vi "putFPGAData.vi"(8 "error in (no error)":errorcluster, 10 "TelemetryFPGAData":T1, 11 "M1M3SAL in":refnum<class "M1M3SAL.lvclass">) -> (0 "error out":errorcluster, 3 "M1M3SAL out":refnum<class "M1M3SAL.lvclass">)   [LabVIEW 2016, in "M1M3SupportCommunicator.lvlib" / "M1M3SAL.lvclass"]
uses:
  M1M3SAL.lvclass
  DataTypes/Topics/TelemetryFPGAData.ctl
  DataTypes/Topics/Parts/Timestamp.ctl
  DataTypes/MessageHeader.ctl
  DataTypes/MessageTypes.ctl
  DataTypes/MessageTopics.ctl
  M1M3SAL.lvclass/M1M3SAL.ctl
  writeU8.vi
  writeI32.vi
  M1M3SupportCommunicator.lvlib
  DataTypes/Topics/M1M3SupportTopics.lvlib
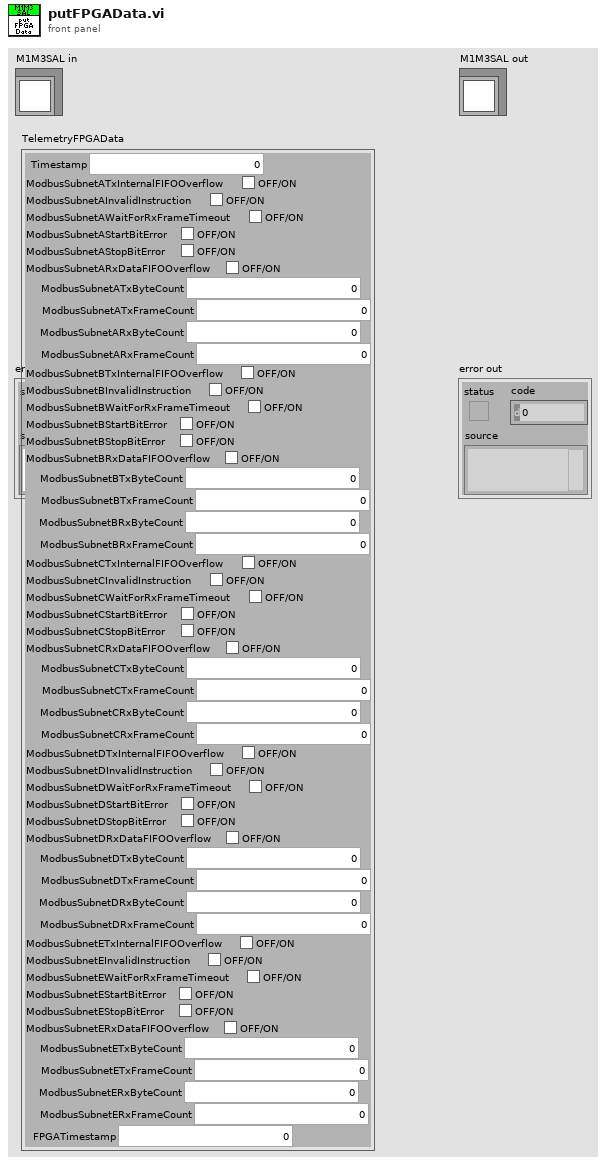
[diagram p1: front panel]
types:
  T1 = typedef "M1M3SupportTopics.lvlib/TelemetryFPGAData.ctl" = cluster{"Timestamp":T2, "ModbusSubnetATxInternalFIFOOverflow":bool, "ModbusSubnetAInvalidInstruction":bool, "ModbusSubnetAWaitForRxFrameTimeout":bool, "ModbusSubnetAStartBitError":bool, "ModbusSubnetAStopBitError":bool, "ModbusSubnetARxDataFIFOOverflow":bool, "ModbusSubnetATxByteCount":u32, "ModbusSubnetATxFrameCount":u32, "ModbusSubnetARxByteCount":u32, "ModbusSubnetARxFrameCount":u32, "ModbusSubnetBTxInternalFIFOOverflow":bool, "ModbusSubnetBInvalidInstruction":bool, "ModbusSubnetBWaitForRxFrameTimeout":bool, "ModbusSubnetBStartBitError":bool, "ModbusSubnetBStopBitError":bool, "ModbusSubnetBRxDataFIFOOverflow":bool, "ModbusSubnetBTxByteCount":u32, "ModbusSubnetBTxFrameCount":u32, "ModbusSubnetBRxByteCount":u32, "ModbusSubnetBRxFrameCount":u32, "ModbusSubnetCTxInternalFIFOOverflow":bool, "ModbusSubnetCInvalidInstruction":bool, "ModbusSubnetCWaitForRxFrameTimeout":bool, "ModbusSubnetCStartBitError":bool, "ModbusSubnetCStopBitError":bool, "ModbusSubnetCRxDataFIFOOverflow":bool, "ModbusSubnetCTxByteCount":u32, "ModbusSubnetCTxFrameCount":u32, "ModbusSubnetCRxByteCount":u32, "ModbusSubnetCRxFrameCount":u32, "ModbusSubnetDTxInternalFIFOOverflow":bool, "ModbusSubnetDInvalidInstruction":bool, "ModbusSubnetDWaitForRxFrameTimeout":bool, "ModbusSubnetDStartBitError":bool, "ModbusSubnetDStopBitError":bool, "ModbusSubnetDRxDataFIFOOverflow":bool, "ModbusSubnetDTxByteCount":u32, "ModbusSubnetDTxFrameCount":u32, "ModbusSubnetDRxByteCount":u32, "ModbusSubnetDRxFrameCount":u32, "ModbusSubnetETxInternalFIFOOverflow":bool, "ModbusSubnetEInvalidInstruction":bool, "ModbusSubnetEWaitForRxFrameTimeout":bool, "ModbusSubnetEStartBitError":bool, "ModbusSubnetEStopBitError":bool, "ModbusSubnetERxDataFIFOOverflow":bool, "ModbusSubnetETxByteCount":u32, "ModbusSubnetETxFrameCount":u32, "ModbusSubnetERxByteCount":u32, "ModbusSubnetERxFrameCount":u32, "FPGATimestamp":dbl}
  T2 = typedef "M1M3SupportTopics.lvlib/Timestamp.ctl" = dbl
  T3 = typedef "M1M3SupportCommunicator.lvlib/MessageHeader.ctl" = cluster{"Type":T4, "Topic":T5, "Size":i32}
  T4 = typedef "M1M3SupportCommunicator.lvlib/MessageTypes.ctl" = enum8{"None", "PutSample", "GetNextSample", "LogEvent", "GetEvent", "IssueCommand", "CommandId", "WaitForCompletion", "AcceptCommand", "AckCommand"}
  T5 = typedef "M1M3SupportCommunicator.lvlib/MessageTopics.ctl" = enum8{"None", "ForceActuatorData", "MirrorForceData", "HardpointData", "AirData", "DynamicData", "FPGAData", "IMSData", "ForceActuatorStatus", "ElevationData", "HardpointStatus", "HardpointActuatorChase", "AirStatus", "ForceActuatorSafetyChecks", "ForceActuatorTest", "ActuatorBroadcastCounter", "StatusChecks", "CellChecks", "HardpointActuatorBreakaway", "RaiseMirrorComplete", "ILCCommunication", "ElevationAngleChecks", "DetailedState", "ServoLoops", "ForceActuatorInfo", "LowerMirrorComplete", "HardpointActuatorInfo", "SettingsApplied", "ErrorCode", "StartupChecks", "SummaryState", "SettingVersions", "ActuatorTestStatus", "AppliedSettingsMatchStart", "Enable", "EnterMaintenance", "Standby", "AbortLowerM1M3", "ApplyAberrationByForces", "ApplyAOSCorrectionByBendingModes", "ClearAOSCorrection", "Start", "RaiseM1M3", "TestForceActuator", "LowerM1M3", "ApplyAOSCorrectionByForces", "Disable", "ApplyAberationByBendingMode", "TestHardpoint", "ManipulateM1M3", "ClearAberration", "Exit", "TestAir", "AbortRaiseM1M3", "MoveHardpointActuators", "ExitMaintenance", "Shutdown"}
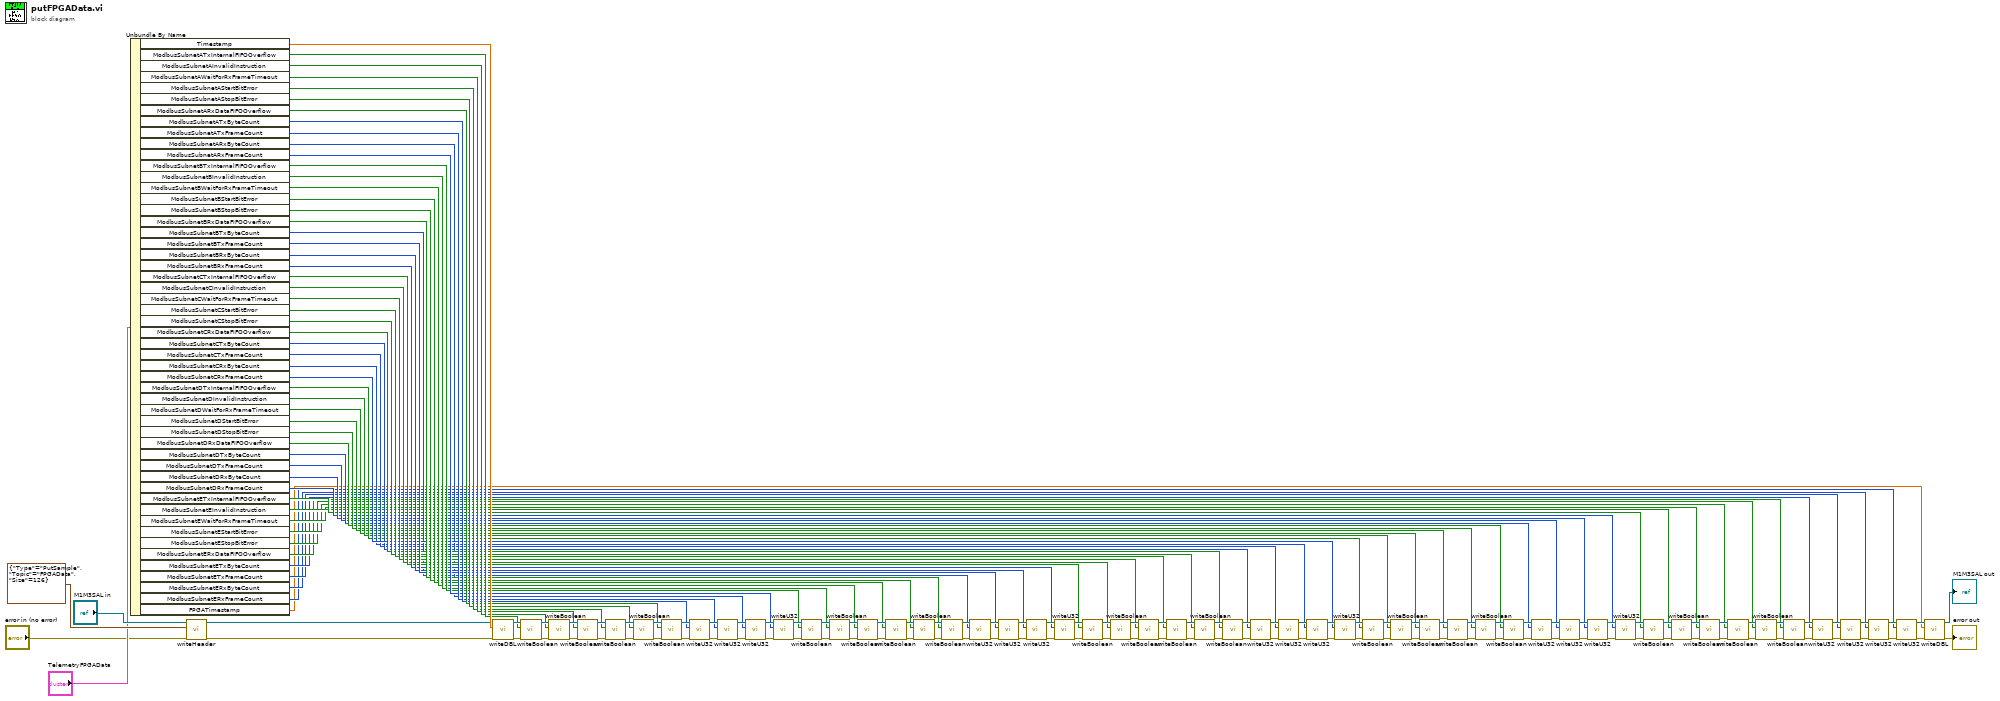
[diagram p0: block diagram]
diagram:
  n1 = Unbundle By Name("TelemetryFPGAData") -> ("Timestamp"=w141:T2, "ModbusSubnetATxInternalFIFOOverflow"=w58:bool, "ModbusSubnetAInvalidInstruction"=w57:bool, "ModbusSubnetAWaitForRxFrameTimeout"=w56:bool, "ModbusSubnetAStartBitError"=w55:bool, "ModbusSubnetAStopBitError"=w54:bool, "ModbusSubnetARxDataFIFOOverflow"=w53:bool, "ModbusSubnetATxByteCount"=w52:u32, "ModbusSubnetATxFrameCount"=w51:u32, "ModbusSubnetARxByteCount"=w33:u32, "ModbusSubnetARxFrameCount"=w50:u32, "ModbusSubnetBTxInternalFIFOOverflow"=w49:bool, "ModbusSubnetBInvalidInstruction"=w48:bool, "ModbusSubnetBWaitForRxFrameTimeout"=w47:bool, "ModbusSubnetBStartBitError"=w46:bool, "ModbusSubnetBStopBitError"=w45:bool, "ModbusSubnetBRxDataFIFOOverflow"=w44:bool, "ModbusSubnetBTxByteCount"=w32:u32, "ModbusSubnetBTxFrameCount"=w43:u32, "ModbusSubnetBRxByteCount"=w42:u32, "ModbusSubnetBRxFrameCount"=w41:u32, "ModbusSubnetCTxInternalFIFOOverflow"=w40:bool, "ModbusSubnetCInvalidInstruction"=w39:bool, "ModbusSubnetCWaitForRxFrameTimeout"=w38:bool, "ModbusSubnetCStartBitError"=w37:bool, "ModbusSubnetCStopBitError"=w36:bool, "ModbusSubnetCRxDataFIFOOverflow"=w35:bool, "ModbusSubnetCTxByteCount"=w31:u32, "ModbusSubnetCTxFrameCount"=w30:u32, "ModbusSubnetCRxByteCount"=w29:u32, "ModbusSubnetCRxFrameCount"=w34:u32, "ModbusSubnetDTxInternalFIFOOverflow"=w28:bool, "ModbusSubnetDInvalidInstruction"=w27:bool, "ModbusSubnetDWaitForRxFrameTimeout"=w26:bool, "ModbusSubnetDStartBitError"=w25:bool, "ModbusSubnetDStopBitError"=w24:bool, "ModbusSubnetDRxDataFIFOOverflow"=w23:bool, "ModbusSubnetDTxByteCount"=w22:u32, "ModbusSubnetDTxFrameCount"=w21:u32, "ModbusSubnetDRxByteCount"=w20:u32, "ModbusSubnetDRxFrameCount"=w19:u32, "ModbusSubnetETxInternalFIFOOverflow"=w18:bool, "ModbusSubnetEInvalidInstruction"=w17:bool, "ModbusSubnetEWaitForRxFrameTimeout"=w16:bool, "ModbusSubnetEStartBitError"=w15:bool, "ModbusSubnetEStopBitError"=w14:bool, "ModbusSubnetERxDataFIFOOverflow"=w13:bool, "ModbusSubnetETxByteCount"=w12:u32, "ModbusSubnetETxFrameCount"=w11:u32, "ModbusSubnetERxByteCount"=w10:u32, "ModbusSubnetERxFrameCount"=w9:u32, "FPGATimestamp"=w7:dbl)
  n2 = call "writeHeader.vi"("error in (no error)"="error in (no error)", "MessageHeader"=T3 {"Type"=enum."PutSample", "Topic"=enum."FPGAData", "Size"=126}, "M1M3SAL in"="M1M3SAL in") -> ("error out"=w4:errorcluster, "M1M3SAL out"=w3:refnum<class "M1M3SAL.lvclass">)  [unwired: 7 in]
  n3 = call "writeDBL.vi"("error in (no error)"=w4, "Input"=w141, "M1M3SAL in"=w3) -> ("error out"=w59:errorcluster, "M1M3SAL out"=w68:refnum<class "M1M3SAL.lvclass">)  [unwired: 7 in]
  n4 = call "writeBoolean.vi"("error in (no error)"=w59, "Input"=w58, "M1M3SAL in"=w68) -> ("error out"=w159:errorcluster, "M1M3SAL out"=w158:refnum<class "M1M3SAL.lvclass">)  [unwired: 7 in]
  n5 = call "writeBoolean.vi"("error in (no error)"=w159, "Input"=w57, "M1M3SAL in"=w158) -> ("error out"=w157:errorcluster, "M1M3SAL out"=w156:refnum<class "M1M3SAL.lvclass">)  [unwired: 7 in]
  n6 = call "writeBoolean.vi"("error in (no error)"=w157, "Input"=w56, "M1M3SAL in"=w156) -> ("error out"=w155:errorcluster, "M1M3SAL out"=w154:refnum<class "M1M3SAL.lvclass">)  [unwired: 7 in]
  n7 = call "writeBoolean.vi"("error in (no error)"=w155, "Input"=w55, "M1M3SAL in"=w154) -> ("error out"=w153:errorcluster, "M1M3SAL out"=w152:refnum<class "M1M3SAL.lvclass">)  [unwired: 7 in]
  n8 = call "writeBoolean.vi"("error in (no error)"=w153, "Input"=w54, "M1M3SAL in"=w152) -> ("error out"=w151:errorcluster, "M1M3SAL out"=w150:refnum<class "M1M3SAL.lvclass">)  [unwired: 7 in]
  n9 = call "writeBoolean.vi"("error in (no error)"=w151, "Input"=w53, "M1M3SAL in"=w150) -> ("error out"=w148:errorcluster, "M1M3SAL out"=w149:refnum<class "M1M3SAL.lvclass">)  [unwired: 7 in]
  n10 = call "writeU32.vi"("error in (no error)"=w148, "Input"=w52, "M1M3SAL in"=w149) -> ("error out"=w147:errorcluster, "M1M3SAL out"=w146:refnum<class "M1M3SAL.lvclass">)  [unwired: 7 in]
  n11 = call "writeU32.vi"("error in (no error)"=w147, "Input"=w51, "M1M3SAL in"=w146) -> ("error out"=w145:errorcluster, "M1M3SAL out"=w144:refnum<class "M1M3SAL.lvclass">)  [unwired: 7 in]
  n12 = call "writeU32.vi"("error in (no error)"=w145, "Input"=w33, "M1M3SAL in"=w144) -> ("error out"=w143:errorcluster, "M1M3SAL out"=w142:refnum<class "M1M3SAL.lvclass">)  [unwired: 7 in]
  n13 = call "writeU32.vi"("error in (no error)"=w143, "Input"=w50, "M1M3SAL in"=w142) -> ("error out"=w66:errorcluster, "M1M3SAL out"=w67:refnum<class "M1M3SAL.lvclass">)  [unwired: 7 in]
  n14 = call "writeBoolean.vi"("error in (no error)"=w66, "Input"=w49, "M1M3SAL in"=w67) -> ("error out"=w123:errorcluster, "M1M3SAL out"=w124:refnum<class "M1M3SAL.lvclass">)  [unwired: 7 in]
  n15 = call "writeBoolean.vi"("error in (no error)"=w123, "Input"=w48, "M1M3SAL in"=w124) -> ("error out"=w125:errorcluster, "M1M3SAL out"=w126:refnum<class "M1M3SAL.lvclass">)  [unwired: 7 in]
  n16 = call "writeBoolean.vi"("error in (no error)"=w125, "Input"=w47, "M1M3SAL in"=w126) -> ("error out"=w127:errorcluster, "M1M3SAL out"=w128:refnum<class "M1M3SAL.lvclass">)  [unwired: 7 in]
  n17 = call "writeBoolean.vi"("error in (no error)"=w127, "Input"=w46, "M1M3SAL in"=w128) -> ("error out"=w129:errorcluster, "M1M3SAL out"=w130:refnum<class "M1M3SAL.lvclass">)  [unwired: 7 in]
  n18 = call "writeBoolean.vi"("error in (no error)"=w129, "Input"=w45, "M1M3SAL in"=w130) -> ("error out"=w131:errorcluster, "M1M3SAL out"=w132:refnum<class "M1M3SAL.lvclass">)  [unwired: 7 in]
  n19 = call "writeBoolean.vi"("error in (no error)"=w131, "Input"=w44, "M1M3SAL in"=w132) -> ("error out"=w134:errorcluster, "M1M3SAL out"=w133:refnum<class "M1M3SAL.lvclass">)  [unwired: 7 in]
  n20 = call "writeU32.vi"("error in (no error)"=w134, "Input"=w32, "M1M3SAL in"=w133) -> ("error out"=w135:errorcluster, "M1M3SAL out"=w136:refnum<class "M1M3SAL.lvclass">)  [unwired: 7 in]
  n21 = call "writeU32.vi"("error in (no error)"=w135, "Input"=w43, "M1M3SAL in"=w136) -> ("error out"=w137:errorcluster, "M1M3SAL out"=w138:refnum<class "M1M3SAL.lvclass">)  [unwired: 7 in]
  n22 = call "writeU32.vi"("error in (no error)"=w137, "Input"=w42, "M1M3SAL in"=w138) -> ("error out"=w139:errorcluster, "M1M3SAL out"=w140:refnum<class "M1M3SAL.lvclass">)  [unwired: 7 in]
  n23 = call "writeU32.vi"("error in (no error)"=w139, "Input"=w41, "M1M3SAL in"=w140) -> ("error out"=w64:errorcluster, "M1M3SAL out"=w65:refnum<class "M1M3SAL.lvclass">)  [unwired: 7 in]
  n24 = call "writeBoolean.vi"("error in (no error)"=w64, "Input"=w40, "M1M3SAL in"=w65) -> ("error out"=w122:errorcluster, "M1M3SAL out"=w121:refnum<class "M1M3SAL.lvclass">)  [unwired: 7 in]
  n25 = call "writeBoolean.vi"("error in (no error)"=w122, "Input"=w39, "M1M3SAL in"=w121) -> ("error out"=w120:errorcluster, "M1M3SAL out"=w119:refnum<class "M1M3SAL.lvclass">)  [unwired: 7 in]
  n26 = call "writeBoolean.vi"("error in (no error)"=w120, "Input"=w38, "M1M3SAL in"=w119) -> ("error out"=w118:errorcluster, "M1M3SAL out"=w117:refnum<class "M1M3SAL.lvclass">)  [unwired: 7 in]
  n27 = call "writeBoolean.vi"("error in (no error)"=w118, "Input"=w37, "M1M3SAL in"=w117) -> ("error out"=w116:errorcluster, "M1M3SAL out"=w115:refnum<class "M1M3SAL.lvclass">)  [unwired: 7 in]
  n28 = call "writeBoolean.vi"("error in (no error)"=w116, "Input"=w36, "M1M3SAL in"=w115) -> ("error out"=w114:errorcluster, "M1M3SAL out"=w113:refnum<class "M1M3SAL.lvclass">)  [unwired: 7 in]
  n29 = call "writeBoolean.vi"("error in (no error)"=w114, "Input"=w35, "M1M3SAL in"=w113) -> ("error out"=w111:errorcluster, "M1M3SAL out"=w112:refnum<class "M1M3SAL.lvclass">)  [unwired: 7 in]
  n30 = call "writeU32.vi"("error in (no error)"=w111, "Input"=w31, "M1M3SAL in"=w112) -> ("error out"=w110:errorcluster, "M1M3SAL out"=w109:refnum<class "M1M3SAL.lvclass">)  [unwired: 7 in]
  n31 = call "writeU32.vi"("error in (no error)"=w110, "Input"=w30, "M1M3SAL in"=w109) -> ("error out"=w108:errorcluster, "M1M3SAL out"=w107:refnum<class "M1M3SAL.lvclass">)  [unwired: 7 in]
  n32 = call "writeU32.vi"("error in (no error)"=w108, "Input"=w29, "M1M3SAL in"=w107) -> ("error out"=w106:errorcluster, "M1M3SAL out"=w105:refnum<class "M1M3SAL.lvclass">)  [unwired: 7 in]
  n33 = call "writeU32.vi"("error in (no error)"=w106, "Input"=w34, "M1M3SAL in"=w105) -> ("error out"=w62:errorcluster, "M1M3SAL out"=w63:refnum<class "M1M3SAL.lvclass">)  [unwired: 7 in]
  n34 = call "writeBoolean.vi"("error in (no error)"=w62, "Input"=w28, "M1M3SAL in"=w63) -> ("error out"=w87:errorcluster, "M1M3SAL out"=w88:refnum<class "M1M3SAL.lvclass">)  [unwired: 7 in]
  n35 = call "writeBoolean.vi"("error in (no error)"=w87, "Input"=w27, "M1M3SAL in"=w88) -> ("error out"=w89:errorcluster, "M1M3SAL out"=w90:refnum<class "M1M3SAL.lvclass">)  [unwired: 7 in]
  n36 = call "writeBoolean.vi"("error in (no error)"=w89, "Input"=w26, "M1M3SAL in"=w90) -> ("error out"=w91:errorcluster, "M1M3SAL out"=w92:refnum<class "M1M3SAL.lvclass">)  [unwired: 7 in]
  n37 = call "writeBoolean.vi"("error in (no error)"=w91, "Input"=w25, "M1M3SAL in"=w92) -> ("error out"=w93:errorcluster, "M1M3SAL out"=w94:refnum<class "M1M3SAL.lvclass">)  [unwired: 7 in]
  n38 = call "writeBoolean.vi"("error in (no error)"=w93, "Input"=w24, "M1M3SAL in"=w94) -> ("error out"=w95:errorcluster, "M1M3SAL out"=w96:refnum<class "M1M3SAL.lvclass">)  [unwired: 7 in]
  n39 = call "writeBoolean.vi"("error in (no error)"=w95, "Input"=w23, "M1M3SAL in"=w96) -> ("error out"=w98:errorcluster, "M1M3SAL out"=w97:refnum<class "M1M3SAL.lvclass">)  [unwired: 7 in]
  n40 = call "writeU32.vi"("error in (no error)"=w98, "Input"=w22, "M1M3SAL in"=w97) -> ("error out"=w99:errorcluster, "M1M3SAL out"=w100:refnum<class "M1M3SAL.lvclass">)  [unwired: 7 in]
  n41 = call "writeU32.vi"("error in (no error)"=w99, "Input"=w21, "M1M3SAL in"=w100) -> ("error out"=w101:errorcluster, "M1M3SAL out"=w102:refnum<class "M1M3SAL.lvclass">)  [unwired: 7 in]
  n42 = call "writeU32.vi"("error in (no error)"=w101, "Input"=w20, "M1M3SAL in"=w102) -> ("error out"=w103:errorcluster, "M1M3SAL out"=w104:refnum<class "M1M3SAL.lvclass">)  [unwired: 7 in]
  n43 = call "writeU32.vi"("error in (no error)"=w103, "Input"=w19, "M1M3SAL in"=w104) -> ("error out"=w60:errorcluster, "M1M3SAL out"=w61:refnum<class "M1M3SAL.lvclass">)  [unwired: 7 in]
  n44 = call "writeBoolean.vi"("error in (no error)"=w60, "Input"=w18, "M1M3SAL in"=w61) -> ("error out"=w86:errorcluster, "M1M3SAL out"=w85:refnum<class "M1M3SAL.lvclass">)  [unwired: 7 in]
  n45 = call "writeBoolean.vi"("error in (no error)"=w86, "Input"=w17, "M1M3SAL in"=w85) -> ("error out"=w84:errorcluster, "M1M3SAL out"=w83:refnum<class "M1M3SAL.lvclass">)  [unwired: 7 in]
  n46 = call "writeBoolean.vi"("error in (no error)"=w84, "Input"=w16, "M1M3SAL in"=w83) -> ("error out"=w82:errorcluster, "M1M3SAL out"=w81:refnum<class "M1M3SAL.lvclass">)  [unwired: 7 in]
  n47 = call "writeBoolean.vi"("error in (no error)"=w82, "Input"=w15, "M1M3SAL in"=w81) -> ("error out"=w80:errorcluster, "M1M3SAL out"=w79:refnum<class "M1M3SAL.lvclass">)  [unwired: 7 in]
  n48 = call "writeBoolean.vi"("error in (no error)"=w80, "Input"=w14, "M1M3SAL in"=w79) -> ("error out"=w78:errorcluster, "M1M3SAL out"=w77:refnum<class "M1M3SAL.lvclass">)  [unwired: 7 in]
  n49 = call "writeBoolean.vi"("error in (no error)"=w78, "Input"=w13, "M1M3SAL in"=w77) -> ("error out"=w75:errorcluster, "M1M3SAL out"=w76:refnum<class "M1M3SAL.lvclass">)  [unwired: 7 in]
  n50 = call "writeU32.vi"("error in (no error)"=w75, "Input"=w12, "M1M3SAL in"=w76) -> ("error out"=w74:errorcluster, "M1M3SAL out"=w73:refnum<class "M1M3SAL.lvclass">)  [unwired: 7 in]
  n51 = call "writeU32.vi"("error in (no error)"=w74, "Input"=w11, "M1M3SAL in"=w73) -> ("error out"=w72:errorcluster, "M1M3SAL out"=w71:refnum<class "M1M3SAL.lvclass">)  [unwired: 7 in]
  n52 = call "writeU32.vi"("error in (no error)"=w72, "Input"=w10, "M1M3SAL in"=w71) -> ("error out"=w70:errorcluster, "M1M3SAL out"=w69:refnum<class "M1M3SAL.lvclass">)  [unwired: 7 in]
  n53 = call "writeU32.vi"("error in (no error)"=w70, "Input"=w9, "M1M3SAL in"=w69) -> ("error out"=w6:errorcluster, "M1M3SAL out"=w8:refnum<class "M1M3SAL.lvclass">)  [unwired: 7 in]
  n54 = call "writeDBL.vi"("error in (no error)"=w6, "Input"=w7, "M1M3SAL in"=w8) -> ("error out"=→"error out":errorcluster, "M1M3SAL out"=→"M1M3SAL out":refnum<class "M1M3SAL.lvclass">)  [unwired: 7 in]
